vi "make_installer.vi"   [LabVIEW 2015, in "lv-bin-7zip.lvlib" / "v1.lvlib"]
uses:
  v1.lvlib
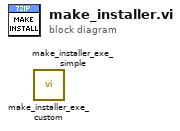
[diagram p0: block diagram]
diagram:
  n1 = call "make_installer_exe_custom.vi"() -> ()  [unwired: 10 in, 2 out]
  n2 = call "make_installer_exe_simple.vi"() -> ()  [unwired: 10 in, 2 out]
